vi "Fetch variable.vi"(11 "Specify location":string) -> (0 "error out":errorcluster, 1 "machine name":string, 2 "Humidity var":refnum<k21>, 3 "Temperature var":refnum<k21>)   [LabVIEW 2016]
uses:
  <vilib>/lvdsc/NI_DSC.lvlib
  <resource>/objmgr/nvio.rc
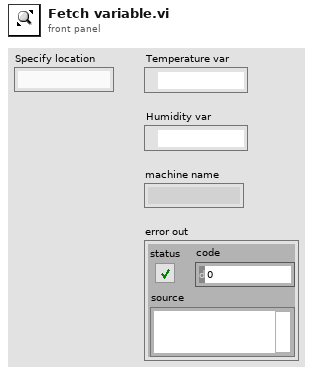
[diagram p1: front panel]
types:
  T1 = cluster{"machine":string, "name":string, "path":path}
  T2 = cluster{"enable? (F)":bool, "data type (deprecated)":enum32{"U32 Bit Field", "Boolean", "Double", "String"}, "log data? (F)":bool, "log alarms & events? (F)":bool, "value resolution (for Float variables only)":dbl, "value deadband (for Float variables only)":dbl, "string logging format (for String variables only)":u32}
  T3 = enum32{"u32BitField", "bool", "double", "string", "int8", "uint8", "int16", "uint16", "int32", "uint32", "int64", "uint64", "single", "double waveform", "int16 waveform", "array of boolean", "array of int8", "array of uint8", "array of int16", "array of uint16", "array of int32", "array of uint32", "array of int64", "array of uint64", "array of single", "array of double", "array of double waveform", "array of int16 waveform", "array of string", "variant", "timestamp", "fixed point", "custom"}
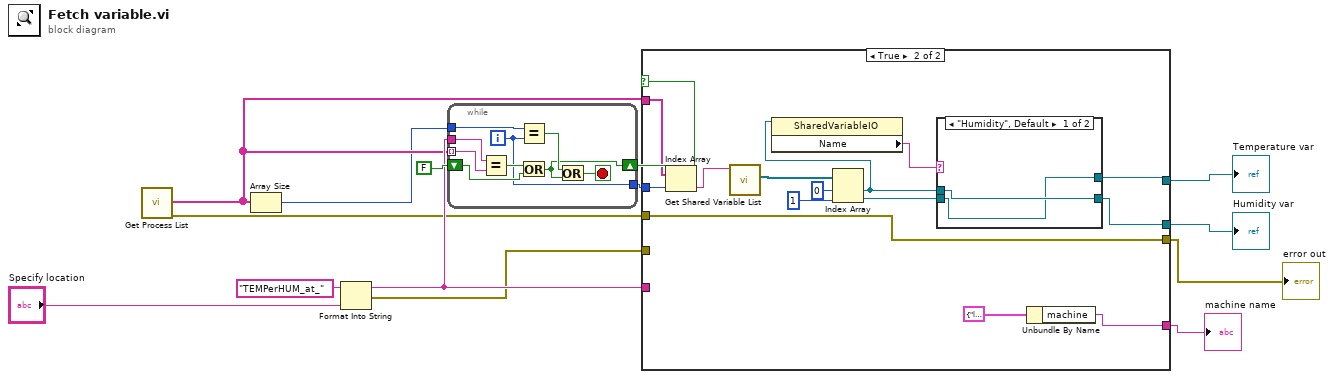
[diagram p0: block diagram]
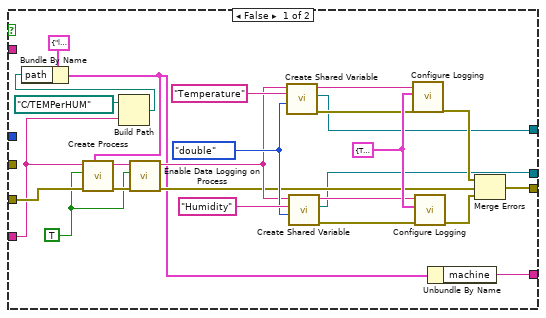
[diagram p2: hidden frame]
diagram:
  n1 = call <vilib>:"Get Process List.vi"() -> ("error out"=w4:errorcluster, "processes"=w3:string[])  [unwired: 10 in]
  n2 = Array Size(array=w3) -> (size(s)=w1:i32)
  n3 = Format Into String(initial string="TEMPerHUM_at_" ("process name"), "Specify location") -> (resulting string=w6:string, error out=w5:errorcluster)  [unwired: 2 in]
  n4 = while {
    tunnel: w3 -> [w23] mode=indexing
    tunnel: w6 -> [w22]
    shift-right: [w16] -> w7
    shift-left: FALSE -> [w20]
    tunnel: [w18] -> w2
    tunnel: w1 -> [w19]
    i -> [w18]
    stop <- w15 stop-if-true
    n5 = Equal?(x=w22, y=w23) -> (x = y?=w21:bool)
    n6 = Equal?(x=w19, y=w18) -> (x = y?=w17:bool)
    n7 = Or(x=w21, y=w20) -> (x .or. y?=w16:bool)
    n8 = Or(x=w17, y=w16) -> (x .or. y?=w15:bool)
  }
  n9 = case shown="True" w7 {
    tunnel: w6 -> [w44 _]
    tunnel: w5 -> [w48 _]
    tunnel: [w28 w62] -> w11
    tunnel: w4 -> [_ w62]
    tunnel: w3 -> [_ w61]
    tunnel: w2 -> [_ w60]
    tunnel: [w27 w51] -> w12
    tunnel: [w26 w49] -> w13
    tunnel: [w24 w54] -> w14
    frame False {
      w36 = T2 {"enable? (F)"=TRUE, "data type (deprecated)"=enum."Double", "log data? (F)"=TRUE, "log alarms & events? (F)"=TRUE, "value resolution (for Float variables only)"=0.0, "value deadband (for Float variables only)"=0.0, "string logging format (for String variables only)"=0} ("logging settings")
      w38 = T3."double" ("data type")
      w41 = TRUE ("run?")
      n10 = Build Path(base path=path "C:/TEMPerHUM", name or relative path=w44) -> (appended path=w45:path)
      n11 = Bundle By Name(cluster=T1 {"machine"="localhost", "name"="Temperature&Humidity", "path"=path "c:/TEMPerHUM"} ("data database"), "path"=w45) -> (w25:T1)
      n12 = call <vilib>:"Create Process.vi"("data database"=w25, "error in (no error)"=w48, "run?"=w41, "process name"=w44) -> ("error out"=w42:errorcluster, "process name out"=w43:string)  [unwired: 6 in]
      n13 = call <vilib>:"Enable Data Logging on Process.vi"("error in (no error)"=w42, "log?"=w41, "process name"=w43) -> ("error out"=w31:errorcluster, "process name out"=w37:string)  [unwired: 7 in]
      n14 = call <vilib>:"Create Shared Variable.vi"("data type"=w38, "shared variable name"="Temperature", "process name"=w37) -> ("error out"=w33:errorcluster, "shared variable"=w27:refnum<k21>, "process name out"=w35:string)  [unwired: 6 in]
      n15 = call <vilib>:"Create Shared Variable.vi"("data type"=w38, "shared variable name"="Humidity", "process name"=w37) -> ("error out"=w32:errorcluster, "shared variable"=w26:refnum<k21>, "process name out"=w34:string)  [unwired: 6 in]
      n16 = call <vilib>:"Configure Logging.vi"("error in (no error)"=w33, "logging settings"=w36, "variable reference in"=w35) -> ("error out"=w30:errorcluster)  [unwired: 7 in, 1 out]
      n17 = call <vilib>:"Configure Logging.vi"("error in (no error)"=w32, "logging settings"=w36, "variable reference in"=w34) -> ("error out"=w29:errorcluster)  [unwired: 7 in, 1 out]
      n18 = Unbundle By Name(w25) -> ("machine"=w24:string)
      n19 = Merge Errors(w30, w31, w29) -> (w28:errorcluster)
    }
    frame True {
      n20 = Index Array(array=w61, index=w60) -> (element=w59:string)
      n21 = call <vilib>:"Get Shared Variable List.vi"("process name"=w59) -> ("shared variables"=w58:refnum<k21>[])  [unwired: 8 in, 2 out]
      n22 = Index Array(array=w58, index #1=0 ("index"), index #2=1 ("index")) -> (element #1=w52:refnum<k21>, element #2=w50:refnum<k21>)
      n23 = property class="SharedVariableIO"(reference=w52) -> ("Name"=w53:string)  [unwired: 1 in, 2 out]
      n24 = case shown="\"Humidity\", Default" w53 {
        tunnel: w52 -> [w64 w66]
        tunnel: [w63 w66] -> w51
        tunnel: w50 -> [w63 w65]
        tunnel: [w64 w65] -> w49
        frame "Humidity", Default {
        }
        frame "Temperature" {
        }
      }
      n25 = Unbundle By Name(T1 {"machine"="localhost", "name"="", "path"=path ""} ("data database")) -> ("machine"=w54:string)
    }
  }
  "machine name" <- w14
  "Humidity var" <- w13
  "Temperature var" <- w12
  "error out" <- w11
